vi "Read.vi"(8 "error in (no error)":errorcluster, 11 "VeriStand DSF in":refnum<class "VeriStand DSF.lvclass">=refnum) -> (0 "error out":errorcluster, 3 "VeriStand DSF out":refnum<class "VeriStand DSF.lvclass">)   [LabVIEW 2017, in "DSF Engine.lvlib" / "VeriStand DSF.lvclass"]
uses:
  VeriStand DSF.lvclass
  DSF Core.lvlibp/Engine/Classes/Framework/Framework.lvclass
  C:/Git/DSF/VeriStand/Data Sharing Custom Device/Source/DSF Core.lvlibp/Engine/Classes/Framework/Framework.lvclass
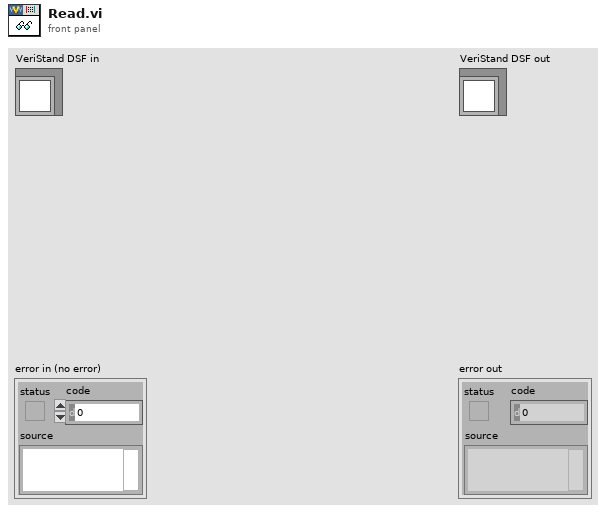
[diagram p1: front panel]
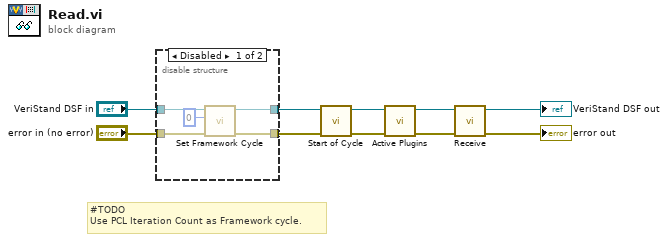
[diagram p0: block diagram]
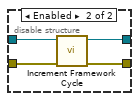
[diagram p2: hidden frame]
diagram:
  # "#TODO\nUse PCL Iteration Count as Framework cycle."
  n1 = disable-structure shown="Disabled" {
    disable-tunnel: "error in (no error)" -> [w15 w18]
    disable-tunnel: "VeriStand DSF in" -> [w14 w19]
    disable-tunnel: [w13 w17] -> w4
    disable-tunnel: [w12 w16] -> w3
    frame Disabled {
      n2 = call "Set Framework Cycle.vi"("error in (no error)"=w15, "iteration"=u64 0, "Framework in"=w14) -> ("error out"=w12:errorcluster, "Framework out"=w13:refnum<class "VeriStand DSF.lvclass">)  [unwired: 7 in]
    }
    frame Enabled {
      n3 = call "Increment Framework Cycle.vi"("error in (no error)"=w18, "Framework in"=w19) -> ("error out"=w16:errorcluster, "Framework out"=w17:refnum<class "VeriStand DSF.lvclass">)  [unwired: 8 in]
    }
  }
  n4 = call "Start of Cycle.vi"("error in (no error)"=w3, "Framework in"=w4) -> ("error out"=w1:errorcluster, "Framework out"=w2:refnum<class "VeriStand DSF.lvclass">)  [unwired: 8 in]
  n5 = call "Active Plugins.vi"("error in (no error)"=w1, "Framework in"=w2) -> ("error out"=w7:errorcluster, "Framework out"=w8:refnum<class "VeriStand DSF.lvclass">)  [unwired: 8 in]
  n6 = call "Receive.vi"("error in (no error)"=w7, "Framework in"=w8) -> ("error out"=→"error out":errorcluster, "Framework out"=→"VeriStand DSF out":refnum<class "VeriStand DSF.lvclass">)  [unwired: 8 in]
